vi "sendData.vi"(2 "error in (no error)":errorcluster, 3 "weight":dbl) -> (0 "error out":errorcluster)   [LabVIEW 2014]
uses:
  <vilib>/httpClient/POSTBuffer.vi
  <vilib>/httpClient/LabVIEWHTTPClient.lvlib
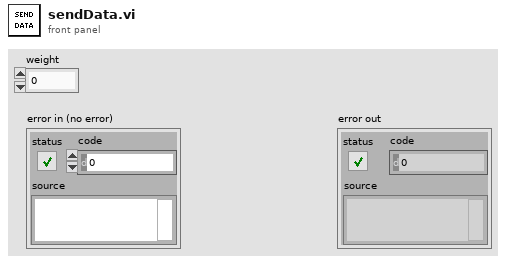
[diagram p1: front panel]
types:
  T1 = typedef "LabVIEWHTTPClient.lvlib/ClientHandle.ctl" = refnum<k1>
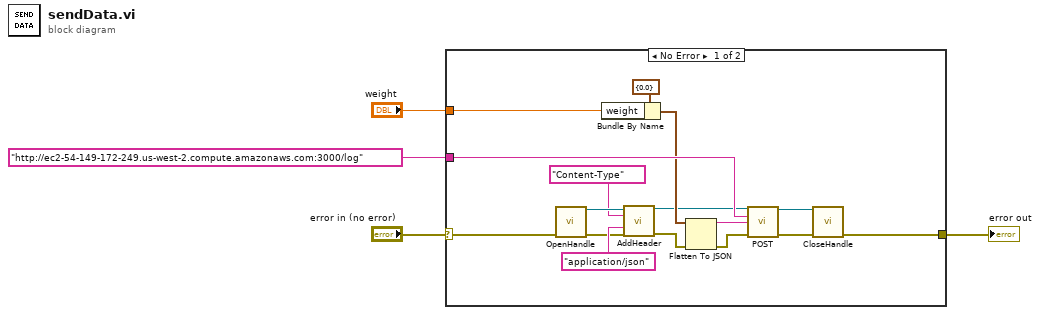
[diagram p0: block diagram]
diagram:
  n1 = case shown="No Error" "error in (no error)" {
    selector: "error in (no error)" -> [w13 w21]
    tunnel: "weight" -> [w8 _]
    tunnel: [w12 w21] -> w2
    tunnel: "http://ec2-54-149-172-249.us-west-2.compute.amazonaws.com:3000/log" ("url") -> [w14 _]
    frame No Error {
      n2 = call <vilib>:"OpenHandle.vi"("error in (no error)"=w13) -> ("client handle out"=w20:T1, "error out"=w17:errorcluster)  [unwired: 13 in]
      n3 = Bundle By Name(cluster=cluster{"weight":dbl} {"weight"=0.0}, "weight"=w8) -> (w7:cluster{"weight":dbl})
      n4 = call <vilib>:"AddHeader.vi"("client handle"=w20, "header"="Content-Type", "value"="application/json", "error in (no error)"=w17) -> ("client handle out"=w5:T1, "error out"=w11:errorcluster)  [unwired: 10 in]
      n5 = Flatten To JSON(anything=w7, error in (no error)=w11) -> (JSON string=w6:string, 11:w10:errorcluster)  [unwired: 1 in]
      n6 = call-poly <vilib>:"POST.vi"("client handle"=w5, "url"=w14, "buffer"=w6, "error in (no error)"=w10) -> ("client handle out"=w16:T1, "error out"=w15:errorcluster)  [unwired: 8 in, 2 out]
      n7 = call <vilib>:"CloseHandle.vi"("client handle"=w16, "error in (no error)"=w15) -> ("error out"=w12:errorcluster)  [unwired: 13 in]
    }
    frame Error {
    }
  }
  "error out" <- w2
